vi "API.vi"(8 "error in (no error)":errorcluster, 11 "DataLogger in":refnum<class "DataLogger.lvclass">) -> (0 "error out":errorcluster, 2 "API":refnum<class "API.lvclass">, 3 "DataLogger out":refnum<class "DataLogger.lvclass">)   [LabVIEW 2020, in "VolatusDataLogger.lvlib" / "DataLogger.lvclass"]
uses:
  DataLogger.lvclass
  C:/Program Files (x86)/National Instruments/LabVIEW 2020/vi.lib/ActorFramework/Actor/Actor.lvclass
  Volatus/API/API.lvclass
  <vilib>/ActorFramework/Actor/Actor.lvclass/Actor.ctl
  <vilib>/ActorFramework/Message Enqueuer/Message Enqueuer.lvclass/Message Enqueuer.ctl
  <vilib>/ActorFramework/Message Enqueuer/Init from Existing Queue.vi
  DataLoggerAPI/DataLoggerAPI.lvclass
  C:/dev/lv20CE/relink/lv-volatus/Volatus/API/API.lvclass
  <vilib>/ActorFramework/Message Enqueuer/Message Enqueuer.lvclass
  DataLogger.lvclass/DataLogger.ctl
  <vilib>/ActorFramework/Actor/Actor.lvclass
  C:/dev/lv20CE/relink/lv-volatus/Volatus/Task/Task.lvclass
  C:/dev/lv20CE/relink/lv-volatus/Volatus/TaskStateHandler/TaskStateHandler.lvclass
  C:/dev/lv20CE/relink/lv-volatus/Volatus/VectoMessageHandler/VectoMessageHandler.lvclass
  C:/dev/lv20CE/relink/lv-volatus/VolatusDataLogger/DataLogger/DataLogger.lvclass
  C:/dev/lv20CE/relink/lv-volatus/Volatus/API Provider/API Provider.lvclass
  C:/dev/lv20CE/relink/lv-volatus/VolatusDataLogger/LoggingHandler/LoggingHandler.lvclass
  C:/dev/lv20CE/relink/lv-volatus/VolatusDataLogger/DataLoggerAPI/DataLoggerAPI.lvclass
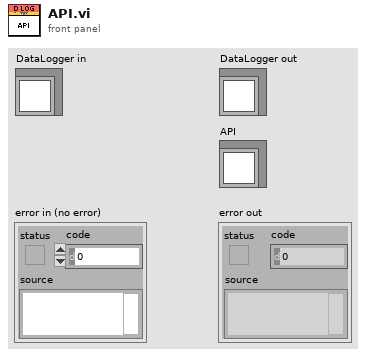
[diagram p1: front panel]
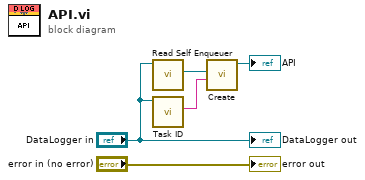
[diagram p0: block diagram]
diagram:
  n1 = call <vilib>:"Read Self Enqueuer.vi"("Actor"="DataLogger in") -> ("Self Enqueuer"=w4:refnum<class "Message Enqueuer.lvclass">)  [unwired: 10 in]
  n2 = call-dynamic "Task ID.vi"("DataLogger in"="DataLogger in") -> ("Task ID"=w2:string)  [unwired: 8 in, 2 out]
  n3 = call "Create.vi"("Task ID"=w2, "EnQr"=w4) -> ("DataLoggerAPI out"=→"API":refnum<class "DataLoggerAPI.lvclass">)  [unwired: 8 in, 1 out]
  "error out" <- "error in (no error)"
  "DataLogger out" <- "DataLogger in"
